vi "WriteVariablesToJSON.vi"(8 "error in":errorcluster, 9 "Channel Values":dbl[](array[numeric]), 10 "Channel Names":string[](array[string]), 11 "path":path) -> (0 "error out":errorcluster, 3 "path out":path)   [LabVIEW 2026]
uses:
  <vilib>/Utility/error.llb/Trim Whitespace (string).vi
  <vilib>/Utility/error.llb/Trim Whitespace One-Sided.vi
panel:
  out "JSON":string
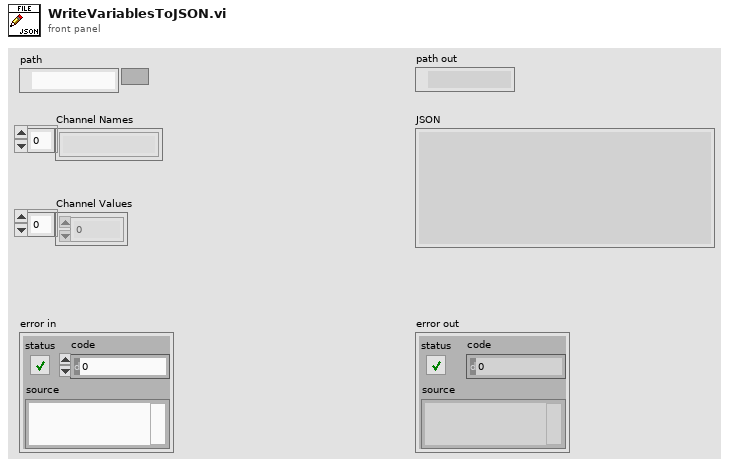
[diagram p1: front panel]
types:
  T1 = enum16{"open", "replace", "create", "open or create", "replace or create", "replace or create with confirmation"}
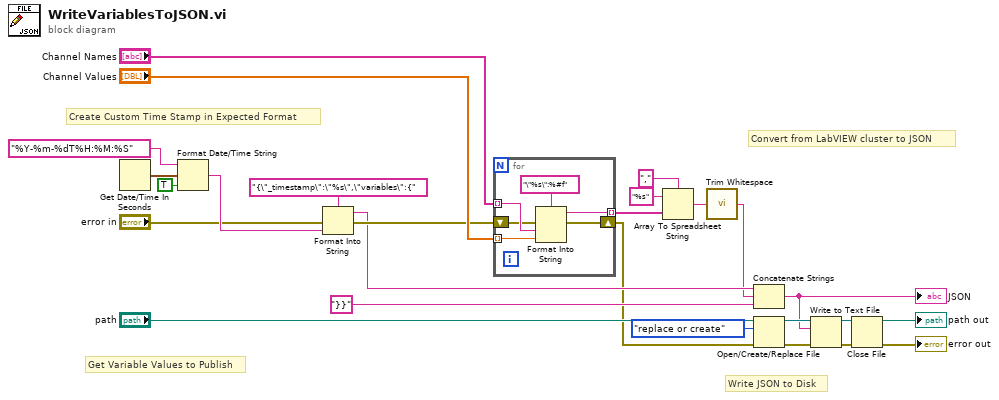
[diagram p0: block diagram]
diagram:
  # "Write JSON to Disk"
  # "Convert from LabVIEW cluster to JSON"
  # "Get Variable Values to Publish"
  # "Create Custom Time Stamp in Expected Format"
  n1 = Get Date/Time In Seconds() -> (seconds since 1Jan1904=w24:timestamp)
  n2 = Format Date/Time String(time format string (%c)="%Y-%m-%dT%H:%M:%S", seconds (now)=w24, UTC format=TRUE) -> (date/time string=w21:string)
  n3 = Format Into String(format string="{\"_timestamp\":\"%s\",\"variables\":{" ("time format string (%c)"), error in="error in", w21) -> (resulting string=w12:string, error out=w17:errorcluster)  [unwired: 1 in]
  n4 = for {
    tunnel: "Channel Names" -> [w31] mode=indexing
    tunnel: "Channel Values" -> [w30] mode=indexing
    shift-right: [w28] -> w1
    shift-left: w17 -> [w29]
    tunnel: [w27] -> w16 mode=indexing
    n5 = Format Into String(format string="\"%s\":%#f" ("time format string (%c)"), error in=w29, w31, w30) -> (resulting string=w27:string, error out=w28:errorcluster)  [unwired: 1 in]
  }
  n6 = Array To Spreadsheet String(delimiter (Tab)=",", array=w16, 3:"%s" ("format string")) -> (spreadsheet string=w11:string)
  n7 = call-poly <vilib>:"Trim Whitespace.vi"("string"=w11) -> ("trimmed string"=w10:string)  [unwired: 1 in]
  n8 = Concatenate Strings(w12, w10, "}}" ("time format string (%c)")) -> (w2:string)
  "JSON" <- w2
  n9 = Open/Create/Replace File(file path (use dialog)="path", error in=w1, operation (0:open)=T1."replace or create") -> (refnum out=w4:refnum<file>, error out=w5:errorcluster)  [unwired: 3 in, 1 out]
  n10 = Write to Text File(file (use dialog)=w4, text=w2, error in=w5) -> (refnum out=w6:refnum<file>, error out=w7:errorcluster)  [unwired: 1 in, 1 out]
  n11 = Close File(refnum=w6, error in=w7) -> (path=→"path out":path, error out=→"error out":errorcluster)
